vi "Hierarchy.vi"() -> (2 "Hierarchy":string)   [LabVIEW 2020, in "ExecAnchor.lvclass"]
uses:
  ExecAnchor.lvclass
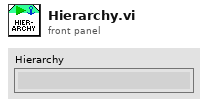
[diagram p1: front panel]
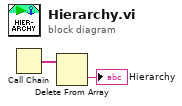
[diagram p0: block diagram]
diagram:
  n1 = Call Chain() -> (call chain=w2:string[])
  n2 = Delete From Array(array=w2) -> (deleted portion=→"Hierarchy":string)  [unwired: 2 in, 1 out]
